vi "CoreGUI.vi"(11 "Cluster":T10) -> ()   [LabVIEW 2024]
uses:
  FileSaver/#SaveFileParameters.ctl
  vision/#AntennaControlNumber.ctl
  <vilib>/userDefined/High Color/IMAQdx.ctl
  dacAquisition/#AquisitionParameter.ctl
  <vilib>/sound2/lvsound2.llb/Sound Data Format.ctl
  Core/#CoreQueues.ctl
  vision/#QueueEnum.ctl
  <vilib>/vision/Image Controls.llb/IMAQ Image.ctl
  #GuiQueueElement.ctl
  #GuiEnum.ctl
  Correlation/#CorrelationQueueElement.ctl
  #GuiState.ctl
panel:
  in  "ResetMeas":bool
  in  "GeneralIndicator":cluster{"StartButton":bool, "StopButton":bool}
  in  "TabControl":T1(tab)
  out "Audio Out":dbl[](graph)
  in  "InSetup":T4={"Proximitor Parameters"={"SampleRate"=10000.0, "BufferSize"=512, "Channels"="cDAQ1Mod1/ai0:3"}, "Output Sound Format"={"sample rate (S/s)"=22050.0, "number of channels"=2, "bits per sample"=16}, "Signal type"=enum."Sine Wave", "Amplitude"=1.0, "Audio Buffer"=0, "Proximitor scaling"=[], "Scalling offset"=0.0} {"Scalling offset" scale=10.0..10000.0; "Amplitude" format="%0.2f"}
  out "Ant4":waveform(dbl)(graph)
  out "Ant3":waveform(dbl)(graph)
  out "Ant2":waveform(dbl)(graph)
  out "Ant1":waveform(dbl)(graph)
  out "DAC DISTANCES":dbl[][](graph)
  out "Image":T5(plugin-control)
  out "FPS":dbl format="%.1f"
  in  "InVision":T8 {"AntDistance [mm]" format="%_6g"}
  out "VISION DISTANCES":dbl[][](graph)
  out "DAC DISTANCES":dbl[][](graph)
  out "Image 2":T5(plugin-control) caption="Image"
  out "Correlation":cluster{dbl[], dbl[]}[](graph)
  out "Image 3":T5(plugin-control) caption="Image"
  out "DAC DISTANCES":dbl[][](graph)
  out "VISION DISTANCES":dbl[][](graph)
  in  "FileSaveParameters":T9
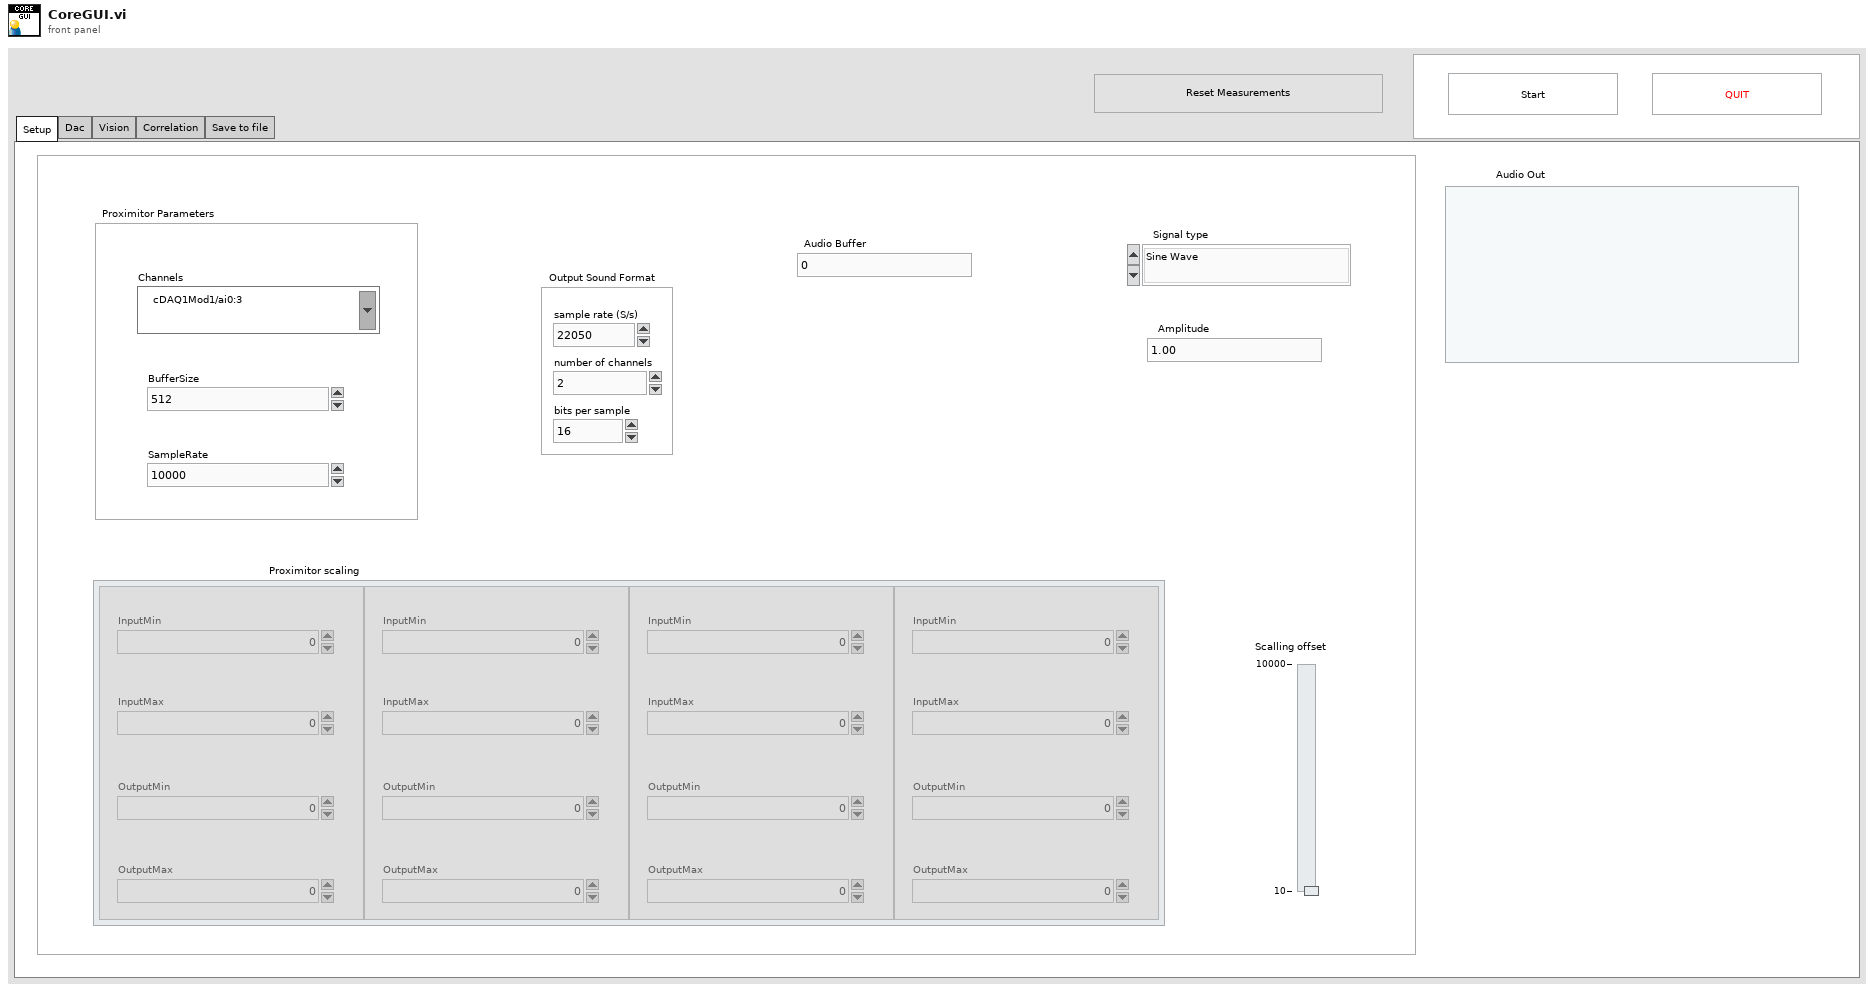
[diagram p1: front panel]
types:
  T1 = enum32{"Setup", "Dac", "Vision", "Correlation", "Save to file"}
  T2 = typedef "#AquisitionParameter.ctl" = cluster{"SampleRate":dbl, "BufferSize":i32, "Channels":tag}
  T3 = typedef "Sound Data Format.ctl" = cluster{"sample rate (S/s)":dbl, "number of channels":i32, "bits per sample":i32}
  T4 = cluster{"Proximitor Parameters":T2, "Output Sound Format":T3, "Signal type":enum16{"Sine Wave", "Triangle Wave", "Square Wave", "Sawtooth Wave"}, "Amplitude":dbl, "Audio Buffer":i32, "Proximitor scaling":cluster{"InputMin":dbl, "InputMax":dbl, "OutputMin":dbl, "OutputMax":dbl}[], "Scalling offset":dbl}
  T5 = typedef "IMAQ Image.ctl" = refnum<image>
  T6 = typedef "#AntennaControlNumber.ctl" = enum16{"Ant1", "Ant2", "Ant3", "Ant4"}
  T7 = typedef "IMAQdx.ctl" = refnum<k21>
  T8 = cluster{"Reverse fingers":bool, "SelectingButton":bool, "Antenna":T6, "TestVsion":bool, "Camera source":T7, "AntDistance [mm]":dbl}
  T9 = typedef "#SaveFileParameters.ctl" = cluster{"StartSaveFile":bool, "TDMS file path":path}
  T10 = typedef "#CoreQueues.ctl" = cluster{"DacData":refnum<queue>, "CorrelationData":refnum<queue>, "VideoData":refnum<queue>, "error out":errorcluster, "ToGUI":refnum<queue>, "FileData":refnum<queue>}
  T11 = typedef "#GuiQueueElement.ctl" = cluster{"Enum":T12, "Variant":variant}
  T12 = typedef "#GuiEnum.ctl" = enum16{"AudioData", "VisionDistances", "DacDistances", "CorrelationDistances", "Video", "DacAquisition", "FPS"}
  T13 = typedef "#GuiState.ctl" = enum16{"Init", "Run", "Close"}
  T14 = cluster{"Global Rectangle":i32[], "Contours":cluster{"Contour Type":u32, "ROI Type":u32, "Points":i32[]}[]}
  T15 = cluster{"Antennas":cluster{"Data":dbl[], "t0":timestamp}, "Video":cluster{"Data":dbl[], "t0":timestamp}}[]
  T16 = cluster{"AquisitionParameters":T2, "SoundFormat":T3, "Signal type":enum16{"Sine Wave", "Triangle Wave", "Square Wave", "Sawtooth Wave"}, "Amplitude":dbl, "AudioBuffer":i32, "ChannelBounds":cluster{"InputMin":dbl, "InputMax":dbl, "OutputMin":dbl, "OutputMax":dbl}[], "MasterOffset":dbl}
  T17 = typedef "NI_Matrix.lvlib/RealMatrix.ctl" = dbl[][]
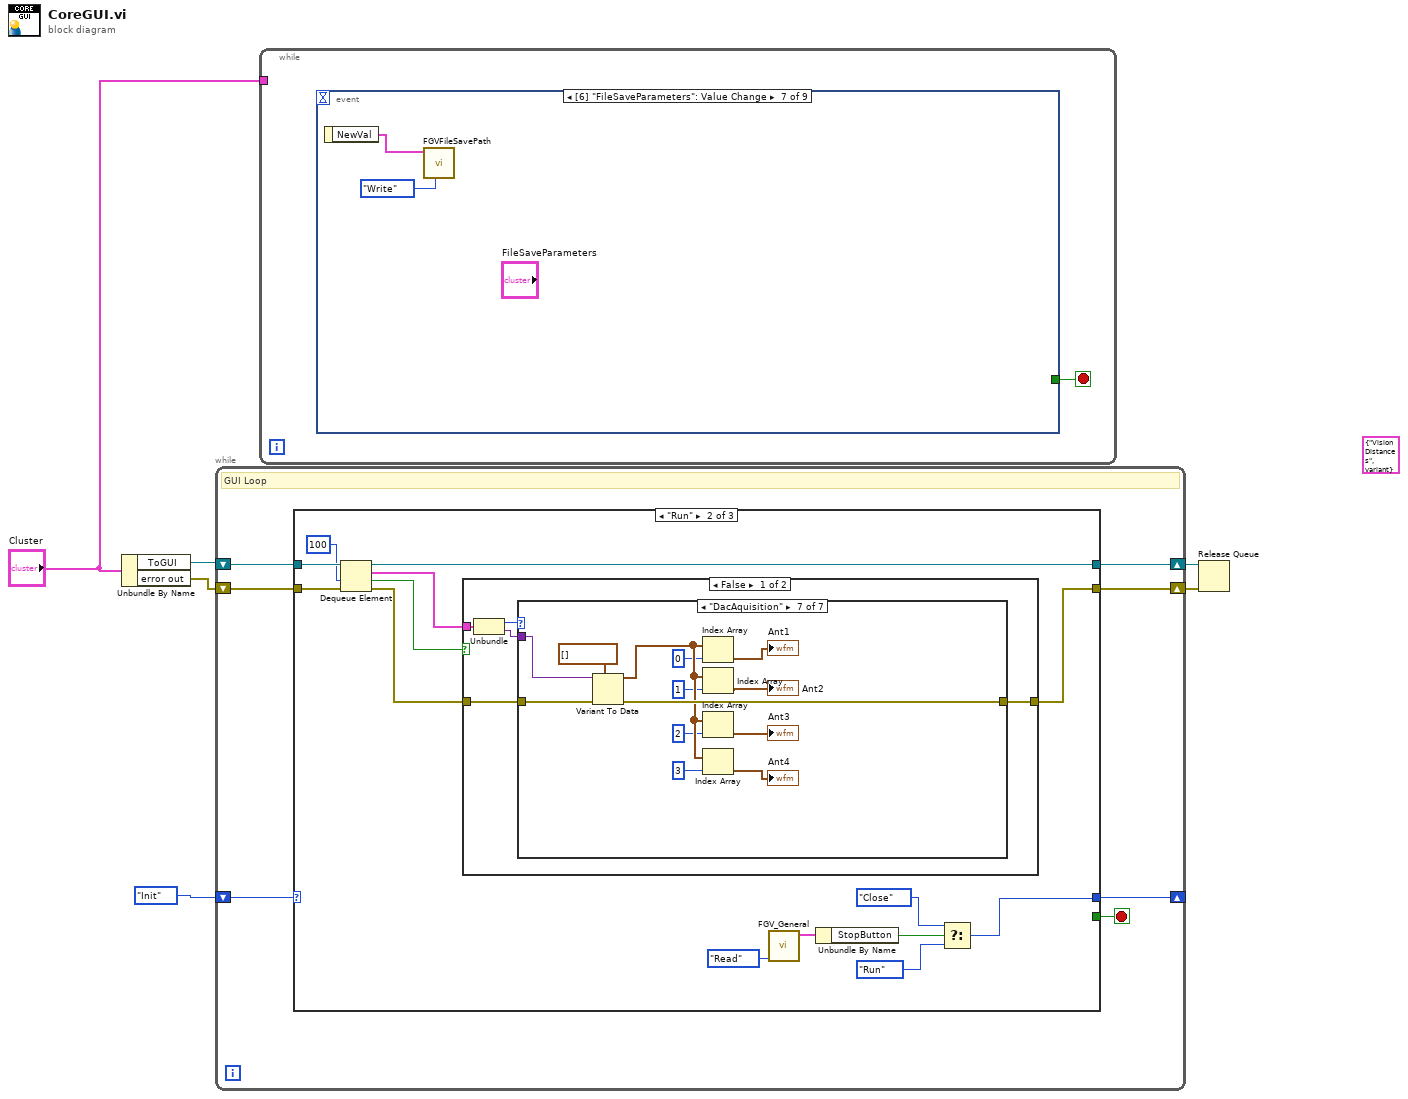
[diagram p0: block diagram]
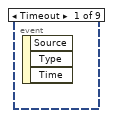
[diagram p2: hidden frame]
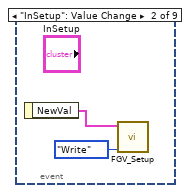
[diagram p3: hidden frame]
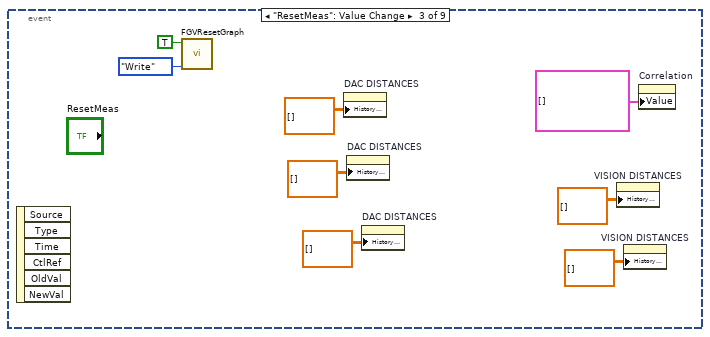
[diagram p4: hidden frame]
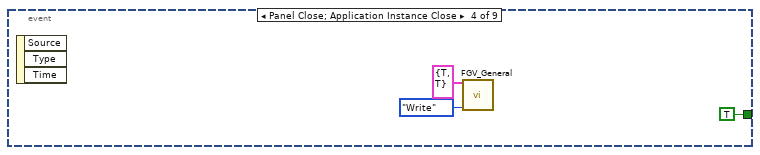
[diagram p5: hidden frame]
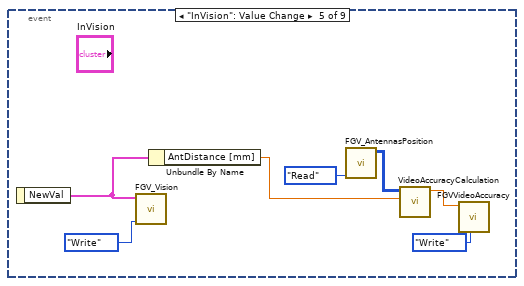
[diagram p6: hidden frame]
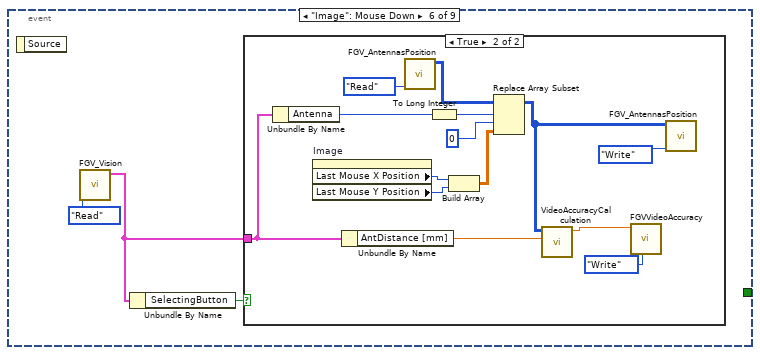
[diagram p7: hidden frame]
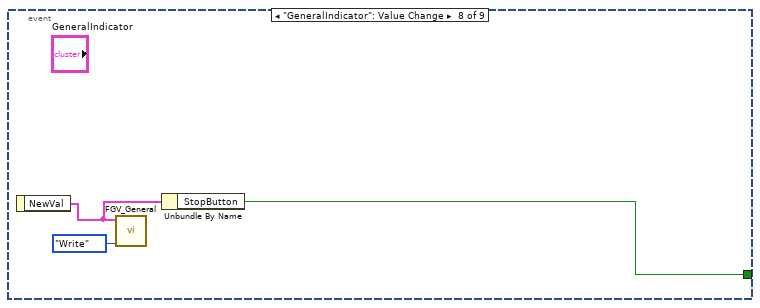
[diagram p9: hidden frame]
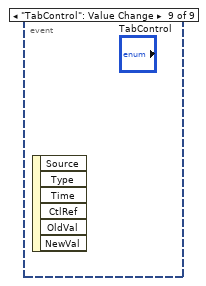
[diagram p10: hidden frame]
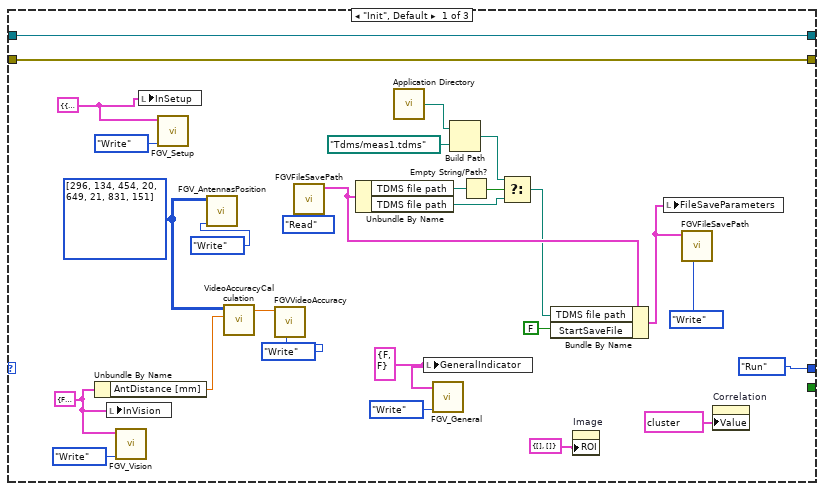
[diagram p11: hidden frame]
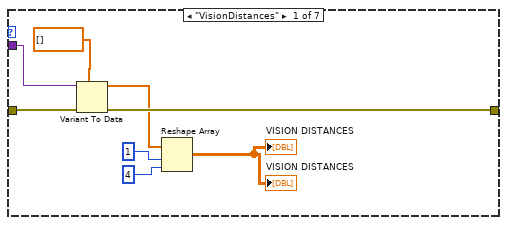
[diagram p12: hidden frame]
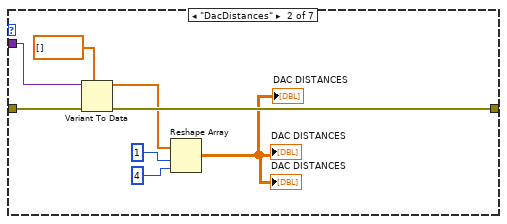
[diagram p13: hidden frame]
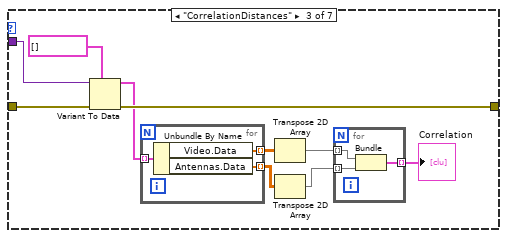
[diagram p14: hidden frame]
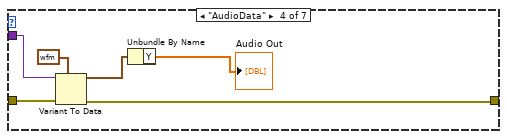
[diagram p15: hidden frame]
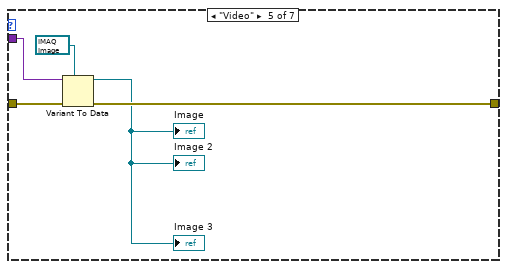
[diagram p16: hidden frame]
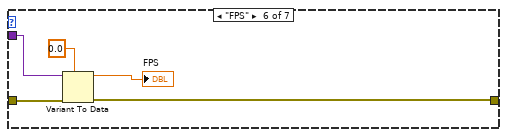
[diagram p17: hidden frame]
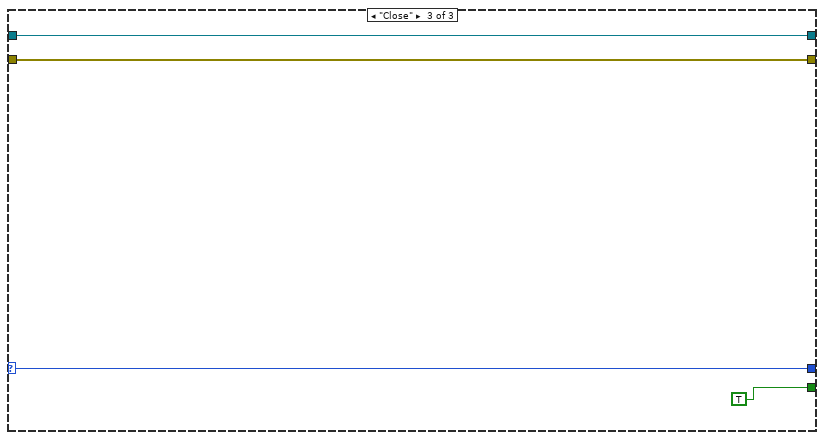
[diagram p19: hidden frame]
diagram:
  (unwired) T11 {"Enum"=enum."VisionDistances", "Variant"=variant} ("element")
  n1 = Unbundle By Name("Cluster") -> ("ToGUI"=w4:refnum<queue>, "error out"=w3:errorcluster)
  n2 = while {
    shift-right: [w11] -> w6
    shift-left: w4 -> [w13]
    shift-right: [w10] -> w5
    shift-left: w3 -> [w12]
    shift-right: [w7] -> _
    shift-left: #GuiState."Init" -> [w9]
    stop <- w8 stop-if-true
    # "GUI Loop"
    n3 = case shown="\"Run\"" w9 {
      selector: w9 -> [_ _ w123]
      tunnel: w13 -> [w41 w55 w126]
      tunnel: w12 -> [w40 w54 w125]
      tunnel: [w41 w53 w126] -> w11
      tunnel: [w40 w49 w125] -> w10
      tunnel: [_ _ TRUE ("StopButton")] -> w8
      tunnel: [#GuiState."Run" w42 w123] -> w7
      frame "Init", Default {
        w24 = cluster{"StartButton":bool, "StopButton":bool} {"StartButton"=FALSE, "StopButton"=FALSE} ("GeneralControl")
        w30 = T8 {"Reverse fingers"=FALSE, "SelectingButton"=FALSE, "Antenna"=enum."Ant1", "TestVsion"=FALSE, "Camera source"="cam1", "AntDistance [mm]"=55.0} ("InVision")
        w32 = u32[][] [[296, 134], [454, 20], [649, 21], [831, 151]] ("AntennasPosition")
        w37 = T16 {"AquisitionParameters"={"SampleRate"=100000.0, "BufferSize"=1000, "Channels"="cDAQ1Mod1/ai0:3"}, "SoundFormat"={"sample rate (S/s)"=22050.0, "number of channels"=2, "bits per sample"=16}, "Signal type"=enum."Triangle Wave", "Amplitude"=1.0, "AudioBuffer"=512, "ChannelBounds"=[{"InputMin"=3000.0, "InputMax"=6000.0, "OutputMin"=100.0, "OutputMax"=400.0}, {"InputMin"=3000.0, "InputMax"=6000.0, "OutputMin"=100.0, "OutputMax"=400.0}, {"InputMin"=3000.0, "InputMax"=6000.0, "OutputMin"=100.0, "OutputMax"=400.0}, {"InputMin"=3000.0, "InputMax"=6000.0, "OutputMin"=100.0, "OutputMax"=400.0}], "MasterOffset"=0.0} ("InSetup")
        n4 = Unbundle By Name(w30) -> ("AntDistance [mm]"=w36:dbl)
        n5 = local write "InVision"(w30) -> ()
        n6 = call "FGV_Vision.vi"("Operation"=enum16{"Read", "Write"}."Write", "InVision"=w30) -> ()  [unwired: 7 in, 1 out]
        n7 = local write "InSetup"(w37) -> ()
        n8 = call "FGV_Setup.vi"("Type"=enum16{"Read", "Write"}."Write", "InSetup"=w37) -> ()  [unwired: 9 in, 1 out]
        n9 = call "FGV_AntennasPosition.vi"("Type"=enum16{"Read", "Write"}."Write", "AntennasPosition"=w32) -> ()  [unwired: 9 in, 1 out]
        n10 = call "VideoAccuracyCalculation.vi"("AntDistance [mm]"=w36, "AntennasPosition"=w32) -> ("VideoAccuracy [mm/px]"=w35:dbl)  [unwired: 9 in]
        n11 = call "FGVVideoAccuracy.vi"("Operation"=enum16{"Read", "Write"}."Write", "VideoAccuracy"=w35) -> ()  [unwired: 9 in, 1 out]
        n12 = call "FGVFileSavePath.vi"("Type"=enum16{"Read", "Write"}."Read") -> ("FileSaveParameters"=w18:T9)  [unwired: 10 in]
        n13 = Unbundle By Name(w18) -> ("TDMS file path"=w23:path, "TDMS file path"=w19:path)
        n14 = call <vilib>:"Application Directory.vi"() -> ("Application Directory"=w14:path)
        n15 = local write "GeneralIndicator"(w24) -> ()
        n16 = call "FGV_General.vi"("Type"=enum16{"Read", "Write"}."Write", "GeneralControl"=w24) -> ()  [unwired: 9 in, 1 out]
        n17 = Build Path(base path=w14, name or relative path=path "Tdms/meas1.tdms") -> (appended path=w20:path)
        n18 = Empty String/Path?(string/path=w23) -> (empty?=w21:bool)
        n19 = Select(t=w20, s=w21, f=w19) -> (s? t:f=w16:path)
        n20 = Bundle By Name(cluster=w18, "TDMS file path"=w16, "StartSaveFile"=FALSE) -> (w15:T9)
        n21 = property on="Image" class="ImageControl"("ROI"=T14 {"Global Rectangle"=[], "Contours"=[]}) -> ()  [unwired: 2 in, 2 out]
        n22 = local write "FileSaveParameters"(w15) -> ()
        n23 = call "FGVFileSavePath.vi"("Type"=enum16{"Read", "Write"}."Write", "FileSaveParameters"=w15) -> ()  [unwired: 9 in, 1 out]
        n24 = property on="Correlation" class="XYGraph (strict)"("Value"=cluster{dbl[], dbl[]}[] [{array[4194 elements], array[4194 elements]}, {array[4194 elements], array[4194 elements]}, {array[4194 elements], array[4194 elements]}, {array[4194 elements], array[4194 elements]}] ("XY Graph")) -> ()  [unwired: 2 in, 2 out]
      }
      frame "Run" {
        n25 = Dequeue Element(queue=w55, timeout in ms (-1)=100, error in (no error)=w54) -> (queue out=w53:refnum<queue>, element=w51:T11, timed out?=w48:bool, error out=w50:errorcluster)
        n26 = case shown="False" w48 {
          tunnel: w51 -> [w60 _]
          tunnel: w50 -> [w57 w122]
          tunnel: [w56 w122] -> w49
          frame False {
            n27 = Unbundle(w60) -> ("Enum"=w59:T12, "Variant"=w58:variant)
            n28 = case shown="\"DacAquisition\"" w59 {
              tunnel: w58 -> [w66 w75 w84 w95 w101 w108 w119]
              tunnel: w57 -> [w68 w74 w86 w97 w103 w107 w121]
              tunnel: [w67 w73 w85 w96 w102 w106 w120] -> w56
              frame "VisionDistances" {
                n29 = Variant To Data(error in=w68, type=dbl[] [] ("output array"), Variant=w66) -> (data=w62:dbl[], error out=w67:errorcluster)
                n30 = Reshape Array(w62, 1 ("dimension size"), 4 ("dimension size")) -> (→"VISION DISTANCES" →"VISION DISTANCES":dbl[][])
              }
              frame "DacDistances" {
                n31 = Variant To Data(error in=w74, type=dbl[] [] ("output array"), Variant=w75) -> (data=w70:dbl[], error out=w73:errorcluster)
                n32 = Reshape Array(w70, 1 ("dimension size"), 4 ("dimension size")) -> (→"DAC DISTANCES" →"DAC DISTANCES" →"DAC DISTANCES":dbl[][])
              }
              frame "CorrelationDistances" {
                n33 = Variant To Data(error in=w86, type=T15 [] ("elements"), Variant=w84) -> (data=w78:T15, error out=w85:errorcluster)
                n34 = for {
                  tunnel: [w92] -> w79 mode=indexing
                  tunnel: [w91] -> w81 mode=indexing
                  tunnel: w78 -> [w90] mode=indexing
                  n35 = Unbundle By Name(w90) -> ("Video.Data"=w92:dbl[], "Antennas.Data"=w91:dbl[])
                }
                n36 = Transpose 2D Array(2D array=w79) -> (transposed array=w82:dbl[][])
                n37 = Transpose 2D Array(2D array=w81) -> (transposed array=w80:dbl[][])
                n38 = for {
                  tunnel: w82 -> [w89] mode=indexing
                  tunnel: w80 -> [w88] mode=indexing
                  tunnel: [w87] -> w77 mode=indexing
                  n39 = Bundle(w89, w88) -> (w87:cluster{dbl[], dbl[]})  [unwired: 1 in]
                }
                "Correlation" <- w77
              }
              frame "AudioData" {
                n40 = Variant To Data(error in=w97, type=waveform(dbl) {"t0"=timestamp(0 s since 1904-01-01), "dt"=1.0, "Y"=[]} ("Output"), Variant=w95) -> (data=w94:waveform(dbl), error out=w96:errorcluster)
                n41 = Unbundle By Name(w94) -> ("Y"=→"Audio Out":dbl[])
              }
              frame "Video" {
                n42 = Variant To Data(error in=w103, type=T5 refnum ("Image"), Variant=w101) -> (data=→"Image" →"Image 3" →"Image 2":T5, error out=w102:errorcluster)
              }
              frame "FPS" {
                n43 = Variant To Data(error in=w107, type=0.0 ("FPS"), Variant=w108) -> (data=→"FPS":dbl, error out=w106:errorcluster)
              }
              frame "DacAquisition" {
                n44 = Variant To Data(error in=w121, type=waveform(dbl)[] [] ("data"), Variant=w119) -> (data=w115:waveform(dbl)[], error out=w120:errorcluster)
                n45 = Index Array(array=w115, index=0) -> (element=→"Ant1":waveform(dbl))
                n46 = Index Array(array=w115, index=1) -> (element=→"Ant2":waveform(dbl))
                n47 = Index Array(array=w115, index=2) -> (element=→"Ant3":waveform(dbl))
                n48 = Index Array(array=w115, index=3) -> (element=→"Ant4":waveform(dbl))
              }
            }
          }
          frame True {
          }
        }
        n49 = call "FGV_General.vi"("Type"=enum16{"Read", "Write"}."Read") -> ("GeneralIndicator"=w46:cluster{"StartButton":bool, "StopButton":bool})  [unwired: 10 in]
        n50 = Unbundle By Name(w46) -> ("StopButton"=w45:bool)
        n51 = Select(t=#GuiState."Close", s=w45, f=#GuiState."Run") -> (s? t:f=w42:T13)
      }
      frame "Close" {
      }
    }
  }
  n52 = while {
    tunnel: "Cluster" -> [_]
    stop <- w127 stop-if-true
    n53 = event shown="[6] \"FileSaveParameters\": Value Change" {
      selector: _ -> [_ _ _ _ _ _ _ _ _]
      dyn-events: _ -> [_ _ _ _ _ _ _ _ _]
      timeout: _ -> [_ _ _ _ _ _ _ _ _]
      tunnel: [_ _ _ TRUE ("StopButton") _ _ _ w168 _] -> w127
      event Timeout {
        n54 = event-data() -> ()  [unwired: 1 in, 3 out]
      }
      event "InSetup": Value Change {
        n55 = event-data() -> ("NewVal"=w128:T4)  [unwired: 1 in]
        n56 = call "FGV_Setup.vi"("Type"=enum16{"Read", "Write"}."Write", "InSetup"=w128) -> ()  [unwired: 9 in, 1 out]
      }
      event "ResetMeas": Value Change {
        n57 = event-data() -> ()  [unwired: 1 in, 6 out]
        n58 = call "FGVResetGraph.vi"("Type"=enum16{"Read", "Write"}."Write", "ResetGraph"=TRUE) -> ()  [unwired: 9 in, 1 out]
        n59 = property on="DAC DISTANCES" class="WFChart (strict)"("History Data"=dbl[][] []) -> ()  [unwired: 2 in, 2 out]
        n60 = property on="DAC DISTANCES" class="WFChart (strict)"("History Data"=dbl[][] []) -> ()  [unwired: 2 in, 2 out]
        n61 = property on="DAC DISTANCES" class="WFChart (strict)"("History Data"=dbl[][] []) -> ()  [unwired: 2 in, 2 out]
        n62 = property on="VISION DISTANCES" class="WFChart (strict)"("History Data"=dbl[][] []) -> ()  [unwired: 2 in, 2 out]
        n63 = property on="VISION DISTANCES" class="WFChart (strict)"("History Data"=dbl[][] []) -> ()  [unwired: 2 in, 2 out]
        n64 = property on="Correlation" class="XYGraph (strict)"("Value"=cluster{dbl[], dbl[]}[] [] ("Correlation")) -> ()  [unwired: 2 in, 2 out]
      }
      event Panel Close; Application Instance Close {
        n65 = event-data() -> ()  [unwired: 1 in, 3 out]
        n66 = call "FGV_General.vi"("Type"=enum16{"Read", "Write"}."Write", "GeneralControl"=cluster{"StartButton":bool, "StopButton":bool} {"StartButton"=TRUE, "StopButton"=TRUE}) -> ()  [unwired: 9 in, 1 out]
      }
      event "InVision": Value Change {
        n67 = event-data() -> ("NewVal"=w143:T8)  [unwired: 1 in]
        n68 = call "FGV_Vision.vi"("Operation"=enum16{"Read", "Write"}."Write", "InVision"=w143) -> ()  [unwired: 7 in, 1 out]
        n69 = Unbundle By Name(w143) -> ("AntDistance [mm]"=w146:dbl)
        n70 = call "FGV_AntennasPosition.vi"("Type"=enum16{"Read", "Write"}."Read") -> ("AntennasPosition"=w141:u32[][])  [unwired: 10 in]
        n71 = call "VideoAccuracyCalculation.vi"("AntDistance [mm]"=w146, "AntennasPosition"=w141) -> ("VideoAccuracy [mm/px]"=w144:dbl)  [unwired: 9 in]
        n72 = call "FGVVideoAccuracy.vi"("Operation"=enum16{"Read", "Write"}."Write", "VideoAccuracy"=w144) -> ()  [unwired: 9 in, 1 out]
      }
      event "Image": Mouse Down {
        n73 = event-data() -> ()  [unwired: 1 in, 1 out]
        n74 = call "FGV_Vision.vi"("Operation"=enum16{"Read", "Write"}."Read") -> ("OutVision"=w150:T8)  [unwired: 8 in]
        n75 = Unbundle By Name(w150) -> ("SelectingButton"=w149:bool)
        n76 = case shown="True" w149 {
          tunnel: w150 -> [_ w157]
          frame False {
          }
          frame True {
            n77 = Unbundle By Name(w157) -> ("Antenna"=w160:T6)
            n78 = property on="Image" class="ImageControl"() -> ("Last Mouse X Position"=w162:i32, "Last Mouse Y Position"=w161:i32)  [unwired: 2 in, 2 out]
            n79 = Unbundle By Name(w157) -> ("AntDistance [mm]"=w159:dbl)
            n80 = call "FGV_AntennasPosition.vi"("Type"=enum16{"Read", "Write"}."Read") -> ("AntennasPosition"=w155:u32[][])  [unwired: 10 in]
            n81 = To Long Integer(number=w160) -> (32bit integer=w164:i32)
            n82 = Build Array(w162, w161) -> (w163:T17)
            n83 = Replace Array Subset(array=w155, new element=w163, index (row)=w164, index (col)=0 ("disabled index (col)")) -> (w153:u32[][])
            n84 = call "VideoAccuracyCalculation.vi"("AntDistance [mm]"=w159, "AntennasPosition"=w153) -> ("VideoAccuracy [mm/px]"=w151:dbl)  [unwired: 9 in]
            n85 = call "FGVVideoAccuracy.vi"("Operation"=enum16{"Read", "Write"}."Write", "VideoAccuracy"=w151) -> ()  [unwired: 9 in, 1 out]
            n86 = call "FGV_AntennasPosition.vi"("Type"=enum16{"Read", "Write"}."Write", "AntennasPosition"=w153) -> ()  [unwired: 9 in, 1 out]
          }
        }
      }
      event Value Change {
        n87 = event-data() -> ("NewVal"=w165:T9)  [unwired: 1 in]
        n88 = call "FGVFileSavePath.vi"("Type"=enum16{"Read", "Write"}."Write", "FileSaveParameters"=w165) -> ()  [unwired: 9 in, 1 out]
      }
      event "GeneralIndicator": Value Change {
        n89 = event-data() -> ("NewVal"=w167:cluster{"StartButton":bool, "StopButton":bool})  [unwired: 1 in]
        n90 = call "FGV_General.vi"("Type"=enum16{"Read", "Write"}."Write", "GeneralControl"=w167) -> ()  [unwired: 9 in, 1 out]
        n91 = Unbundle By Name(w167) -> ("StopButton"=w168:bool)
      }
      event "TabControl": Value Change {
        n92 = event-data() -> ()  [unwired: 1 in, 6 out]
      }
    }
  }
  n93 = Release Queue(queue=w6, error in (no error)=w5) -> ()  [unwired: 1 in, 3 out]
